vi "Failure Message.vi"() -> ()   [LabVIEW 2017, in "Transparent Assertions.Tests.lvlib" / "Assert Not In Range.lvlib"]
uses:
  Assert Not In Range.lvlib
  src/Transparent Assertions/Transparent Assertions.lvlib
panel:
  out "error out":errorcluster
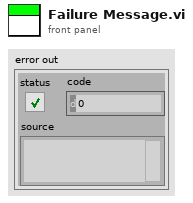
[diagram p1: front panel]
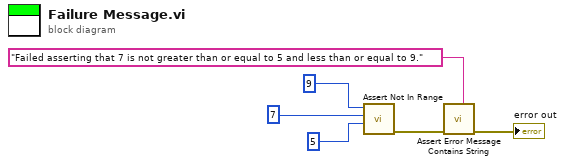
[diagram p0: block diagram]
diagram:
  n1 = call "Assert Not In Range.vi"("Minimum"=5, "Actual"=7, "Maximum"=9) -> ("error out"=w2:errorcluster)  [unwired: 8 in]
  n2 = call "Assert Error Message Contains String.vi"("Expected"="Failed asserting that 7 is not greater than or equal to 5 and less than or equal to 9.", "error in (no error)"=w2) -> ("error out"=→"error out":errorcluster)  [unwired: 9 in]
